vi "Active Power.vi"(4 "Current Waveform":dbl[](array[numeric]), 5 "Voltage Waveform":dbl[](array[numeric])) -> (1 "Active Power":dbl)   [LabVIEW 2014]
uses:
  <vilib>/Analysis/3filter.llb/Filter Passband Type.ctl
  <vilib>/Analysis/NI_AALPro.lvlib
  <vilib>/ptbypt/NI_PtbyPt.lvlib
  <vilib>/Analysis/NI_AALBase.lvlib
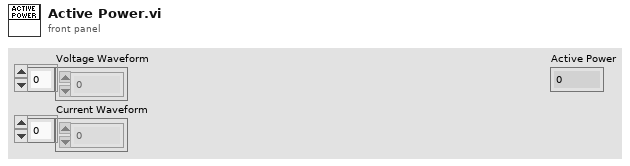
[diagram p1: front panel]
types:
  T1 = typedef "NI_AALBase.lvlib/Filter Passband Type.ctl" = enum32{"Lowpass", "Highpass", "Bandpass", "Bandstop"}
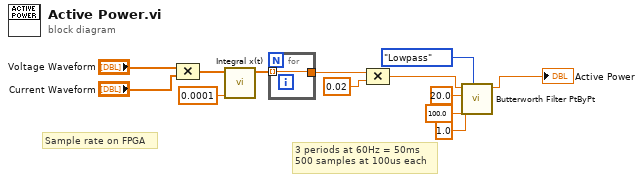
[diagram p0: block diagram]
diagram:
  # "Sample rate on FPGA"
  # "3 periods at 60Hz = 50ms\n500 samples at 100us each"
  n1 = Compound Arithmetic op=MULTIPLY("Voltage Waveform", "Current Waveform") -> (w9:dbl[])
  n2 = call <vilib>:"Integral x(t).vi"("dt"=0.0001, "X"=w9) -> ("Integral X"=w13:dbl[])  [unwired: 8 in, 1 out]
  n3 = for {
    tunnel: w13 -> [w14] mode=indexing
    tunnel: [w14] -> w11
  }
  n4 = Compound Arithmetic op=MULTIPLY(w11, 0.02 ("dt")) -> (w6:dbl)
  n5 = call <vilib>:"Butterworth Filter PtByPt.vi"("filter type"=Filter_Passband_Type."Lowpass", "low cutoff freq: fl"=1.0, "high cutoff freq: fh"=100.0, "sampling freq: fs"=20.0, "x"=w6) -> ("Filtered x"=→"Active Power":dbl)  [unwired: 4 in, 1 out]
